vi "shiftlever.vi"() -> ()   [LabVIEW 2015]
uses:
  <vilib>/myRIO/Instrument Drivers/Onboard IO/AO/AO.lvlib
  rio_Global.vi
panel:
  out "error out":errorcluster
  in  "updown (A/AO1 (Pin 4))":dbl
  in  "leftright (A/AO0 (Pin 2))":dbl
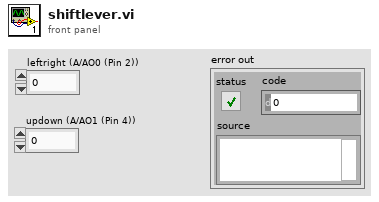
[diagram p1: front panel]
types:
  T1 = typedef "AO.lvlib/AO Reference.ctl" = cluster{"myRIO Reference":T2, "AO Channel List":T6, "AO Scaling Constant List":T8}
  T2 = typedef "myRIO Generic Hardware Reference.ctl" = cluster{"myRIO Model":T3, "myRIO Hardware Reference":T4}
  T3 = typedef "Hardware Version Enum.ctl" = enum16{"Unknown", "myRIO-1900", "myRIO-1950", "roboRIO"}
  T4 = typedef "myRIO v1.0 Reference.ctl" = cluster{"Generic FPGA Reference":T5, "Allow multiple opens":bool}
  T5 = typedef "Generic FPGA Reference.ctl" = refnum<k20>
  T6 = typedef "AO Channels List.ctl" = T7[]
  T7 = typedef "AO Channels Enum.ctl" = enum16{"Not Connected", "AudioOut/Left", "AudioOut/Right", "C/AO0", "C/AO1", "A/AO0", "A/AO1", "B/AO0", "B/AO1"}
  T8 = typedef "Analog Scaling Constants List.ctl" = T9[]
  T9 = typedef "Analog Scaling Constants.ctl" = cluster{"LSB Weight (Volts)":dbl, "Offset (Volts)":dbl, "Signed?":bool}
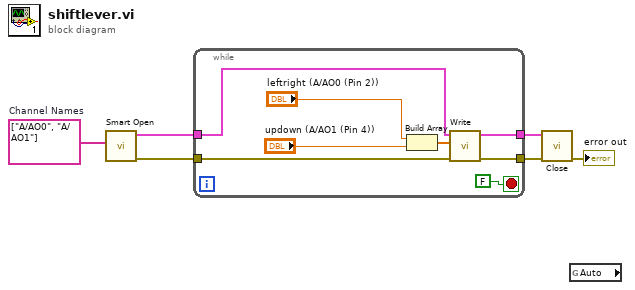
[diagram p0: block diagram]
diagram:
  w6 = tag[] ["A/AO0", "A/AO1"]  # Channel Names
  n1 = call <vilib>:"Smart Open.vi"("Channel Names"=w6) -> ("error out"=w4:errorcluster, "AO Ref Out"=w5:T1)  [unwired: 9 in]
  n2 = while {
    tunnel: w5 -> [w11]
    tunnel: w4 -> [w10]
    tunnel: [w9] -> w2
    tunnel: [w7] -> w3
    stop <- FALSE stop-if-true
    n3 = Build Array("leftright (A/AO0 (Pin 2))", "updown (A/AO1 (Pin 4))") -> (w14:dbl[])
    n4 = call <vilib>:"Write.vi"("error in (no error)"=w10, "Values"=w14, "AO Ref In"=w11) -> ("error out"=w9:errorcluster, "AO Ref Out"=w7:T1)  [unwired: 6 in]
  }
  n5 = call <vilib>:"Close.vi"("error in (no error)"=w2, "AO Ref In"=w3) -> ("error out"=→"error out":errorcluster)  [unwired: 9 in]
  n6 = global read "rio_Global.vi" "Auto"() -> ()  [unwired: 1 out]
